vi "To Generic.vi"(8 "error in (no error)":errorcluster, 11 "Instrument Error Data in":refnum<class "Instrument Data.lvclass">) -> (0 "error out":errorcluster, 2 "Generic Data":refnum<class "Generic Data.lvclass">[](array[class]), 3 "Data Name":string[](array[string]))   [LabVIEW 2020, in "Instrument Handler.lvlib" / "Instrument Data.lvclass"]
doc: "Present private data as an array of named generic data elements."
uses:
  Instrument Data.lvclass
  PPL/HDH.Data.Generic.lvlibp/Generic Data/Generic Data.lvclass
  Instrument Data.lvclass/Instrument Data.ctl
  PPL/HDH.Data.Generic.lvlibp/Generic Data/U32/U32.lvclass
  C:/Current projects/WS/PPL/HDH.Data.Generic.lvlibp/Generic Data/Generic Data.lvclass
  PPL/HDH.Actor Framework.Core.Publisher.lvlibp/Messages/Timed Msg/Data/Timed Data/Timed Data.lvclass
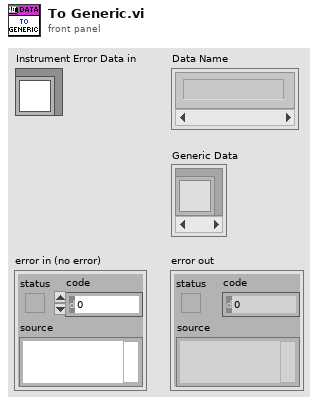
[diagram p1: front panel]
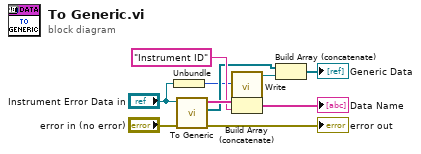
[diagram p0: block diagram]
diagram:
  n1 = Unbundle("Instrument Error Data in") -> (w2:u32)
  n2 = call-parent "To Generic.vi"("error in (no error)"="error in (no error)", "Request Data in"="Instrument Error Data in") -> ("error out"=→"error out":errorcluster, "Generic Data"=w5:refnum<class "Generic Data.lvclass">[], "Data Name"=w8:string[])  [unwired: 7 in]
  n3 = call "Write.vi"("U32"=w2) -> ("U32 out"=w3:refnum<class "U32.lvclass">)  [unwired: 10 in]
  n4 = Build Array (concatenate)(w8, "Instrument ID" ("array")) -> (→"Data Name":string[])
  n5 = Build Array (concatenate)(w5, w3) -> (→"Generic Data":refnum<class "Generic Data.lvclass">[])
